vi "Factorial.vi"() -> ()   [LabVIEW 2014]
panel:
  out "Numeric 2":dbl
  in  "Numeric":i32
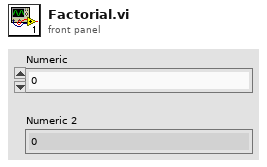
[diagram p1: front panel]
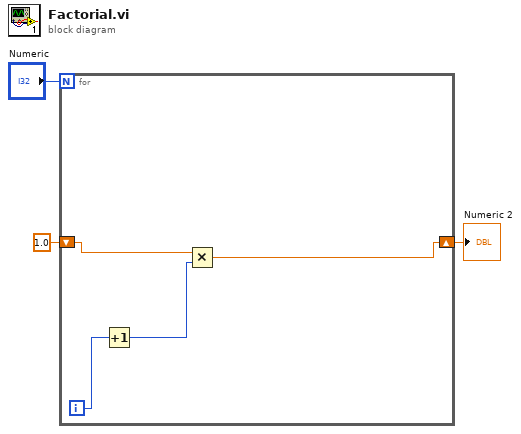
[diagram p0: block diagram]
diagram:
  n1 = for {
    N: "Numeric" -> [_]
    shift-right: [w7] -> w1
    shift-left: 1.0 -> [w6]
    i -> [w5]
    n2 = Increment(x=w5) -> (x+1=w4:i32)
    n3 = Multiply(x=w6, y=w4) -> (x*y=w7:dbl)
  }
  "Numeric 2" <- w1
